vi "Launch Controller.vi"(8 "error in":errorcluster) -> ()   [LabVIEW 2016]
doc: "This VI executes continuously carrying out the current operation and responding to updates or new operations. It will often contain the timing or control code that is difficult to place directly in TeleOp. This VI generally opens all sensors and motors and isolates the rest of the robot code from knowing how the operations are carried out."
uses:
  Launch Setpoints.ctl
  Launch Operations.ctl
  <vilib>/Platform/TimedLoop/XDataNode/timing_clust.ctl
  <vilib>/Platform/TimedLoop/XDataNode/nitl_modes.ctl
  <vilib>/Platform/TimedLoop/XDataNode/wakeup.ctl
  <vilib>/Rock Robotics/Network Tables/NT Write Boolean.vi
  <vilib>/Rock Robotics/Network Tables/NT Read Boolean.vi
  <vilib>/Rock Robotics/Network Tables/NT Read Number.vi
  <vilib>/Platform/TimedLoop/XDataNode/XDataNode.xnode
  <vilib>/Platform/TimedLoop/XDataNode/XDNodeRunTimeDep.lvlib
panel:
  out "Launcher RPM":dbl=3319.8279051826034
  out "Feeder RPM":dbl=3319.8279051826034
  out "Current\nCmd":string
  # "Tip: It may be helpful to observe inputs and sensor values.\nYou may also want to display tuning or debugging controls."
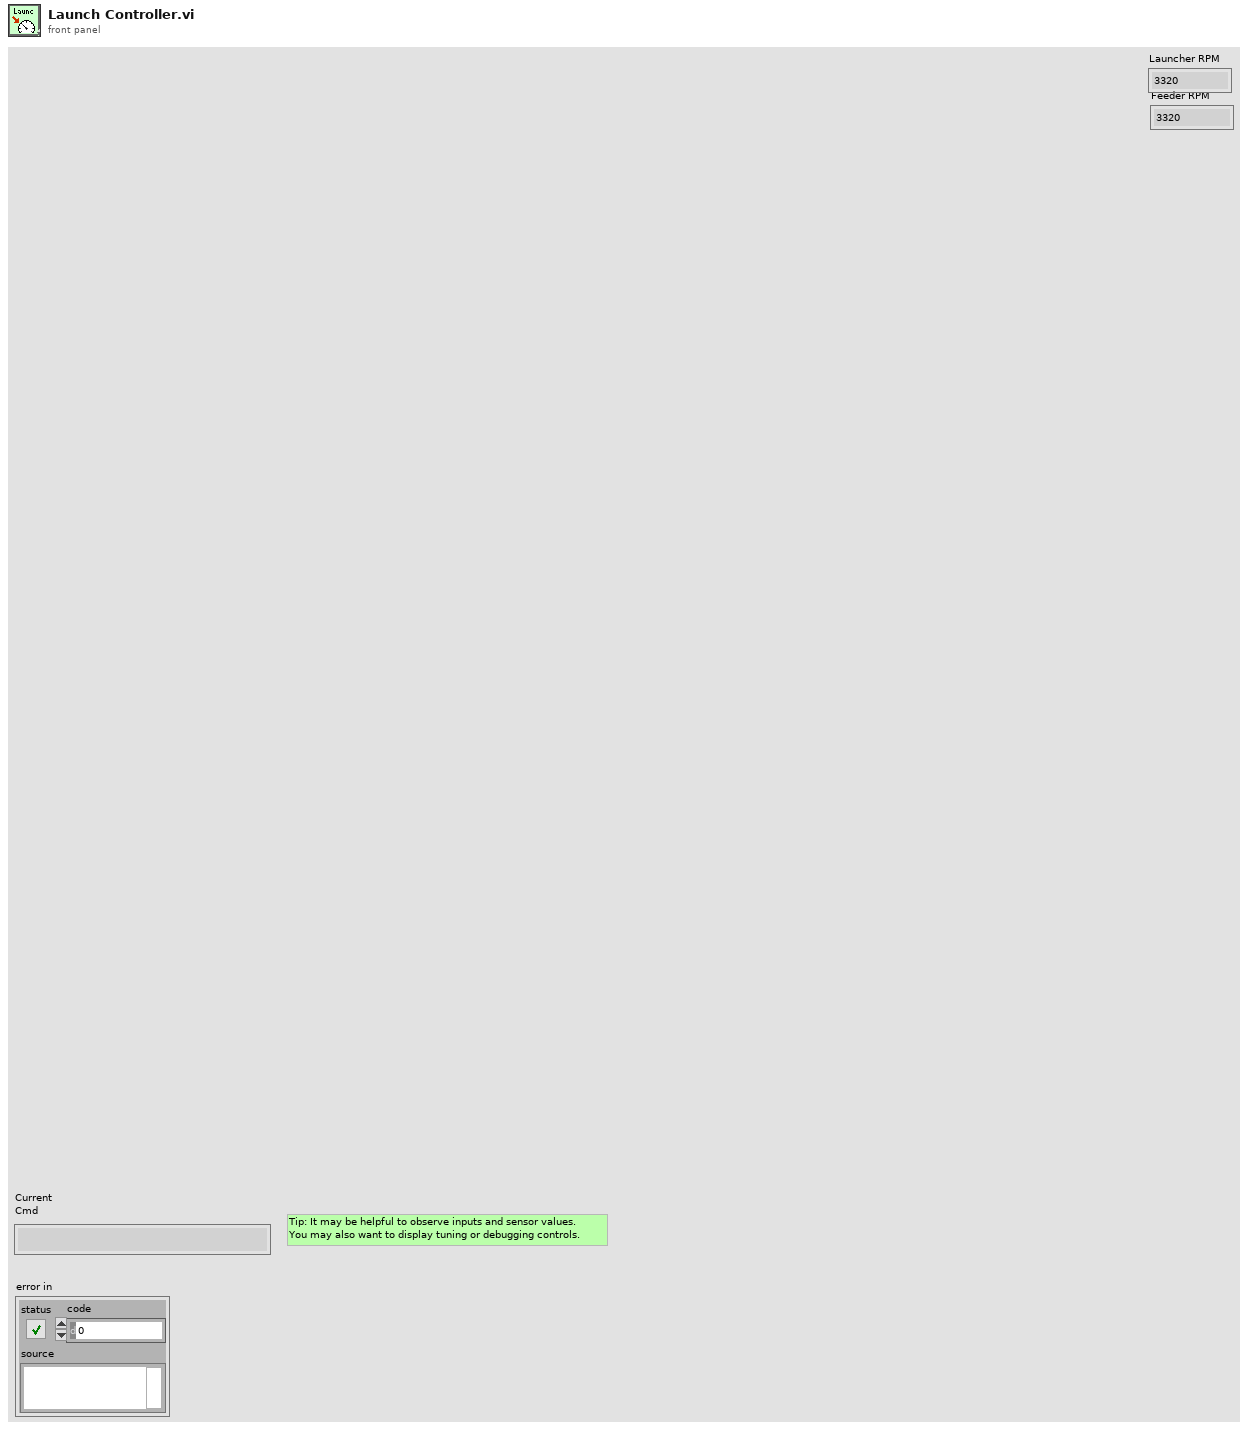
[diagram p1: front panel]
types:
  T1 = typedef "Launch Setpoints.ctl" = cluster{"Operation":T2, "Setpoint":dbl, "Duration":dbl}
  T2 = typedef "Launch Operations.ctl" = enum16{"Reserve", "Read Current", "Immediate", "Set Adgitator", "Toggle Launcher"}
  T3 = typedef "XDNodeRunTimeDep.lvlib/timing_clust.ctl" = cluster{"Expected End [f-1]":u64, "Actual End [f-1]":u64, "Finished Late? [f-1]":bool, "Expected End [i-1]":u64, "Actual End [i-1]":u64, "Finished Late? [i-1]":bool, "Expected Start [i]":u64, "Actual Start [i]":u64, "Expected Start [f]":u64, "Actual Start [f]":u64, "Source Name":string, "Structure Name":string, "Period":i64, "Deadline":i64, "Offset":i64, "Start":i64, "Priority":i32, "Timeout":i32, "Mode":T4, "Wakeup Reason":T5, "Error":errorcluster, "Source Type":string, "Secondary Source Type":string, "Global End Time":u64, "Global Start Time":u64, "Frame Duration":u64, "Iteration Duration":u64, "Assigned CPU":i32, "I/O Scan Engine Mode":u32}
  T4 = typedef "XDNodeRunTimeDep.lvlib/nitl_modes.ctl" = enum32{"No Change", "Process missed periods, maintain original phase", "Discard missed periods, maintain original phase", "Process missed periods, ignore original phase", "Discard missed periods, ignore original phase"}
  T5 = typedef "XDNodeRunTimeDep.lvlib/wakeup.ctl" = enum32{"Normal", "Aborted", "Asynchronous wakeup", "Timing source error", "Timed loop error", "Timeout"}
  T6 = typedef "WPI_MotorControlDeviceRef.ctl" = cluster{"DeviceStatus":errorcluster, "Type":T7, "PWM":cluster{"PWM Channel":T8, "DeadBand":T9}, "CAN":cluster{"Device Number":u8, "SetOutput VI Ref":variant, "GetOutput VI Ref":variant, "Enable VI Ref":variant, "Disable VI Ref":variant, "Data":variant}, "Invert":bool}
  T7 = typedef "WPI_MotorControlType.ctl" = enum16{"PWM", "CAN"}
  T8 = typedef "FPGA_DIOPWMChannel.ctl" = enum8{"PWM 0", "PWM 1", "PWM 2", "PWM 3", "PWM 4", "PWM 5", "PWM 6", "PWM 7", "PWM 8", "PWM 9", "PWM MXP 0", "PWM MXP 1", "PWM MXP 2", "PWM MXP 3", "PWM MXP 4", "PWM MXP 5", "PWM MXP 6", "PWM MXP 7", "PWM MXP 8", "PWM MXP 9", "Invalid"}
  T9 = typedef "WPI_PWMDeadband.ctl" = cluster{"Name":string, "maxPositivePwm":i32, "minPositivePwm":i32, "centerPwm":i32, "maxNegativePwm":i32, "minNegativePwm":i32, "angularRange":u16}
  T10 = typedef "Command Status Info.ctl" = cluster{"Name":string, "Status":T11, "notifier out":T12}
  T11 = typedef "Completion Status.ctl" = enum16{"Successful", "Aborted", "Incomplete"}
  T12 = typedef "Completion Notifier.ctl" = refnum<notifier>
  T13 = cluster{"Default Command":T1, "Command Timing":cluster{"Start Time (ms)":u32, "Iterations":i32}, "Command Arguments":cluster{"Command Info":T10, "Description":string, "Default Command":T1, "notifier out":refnum<notifier>, "Subsystem Name":string}}
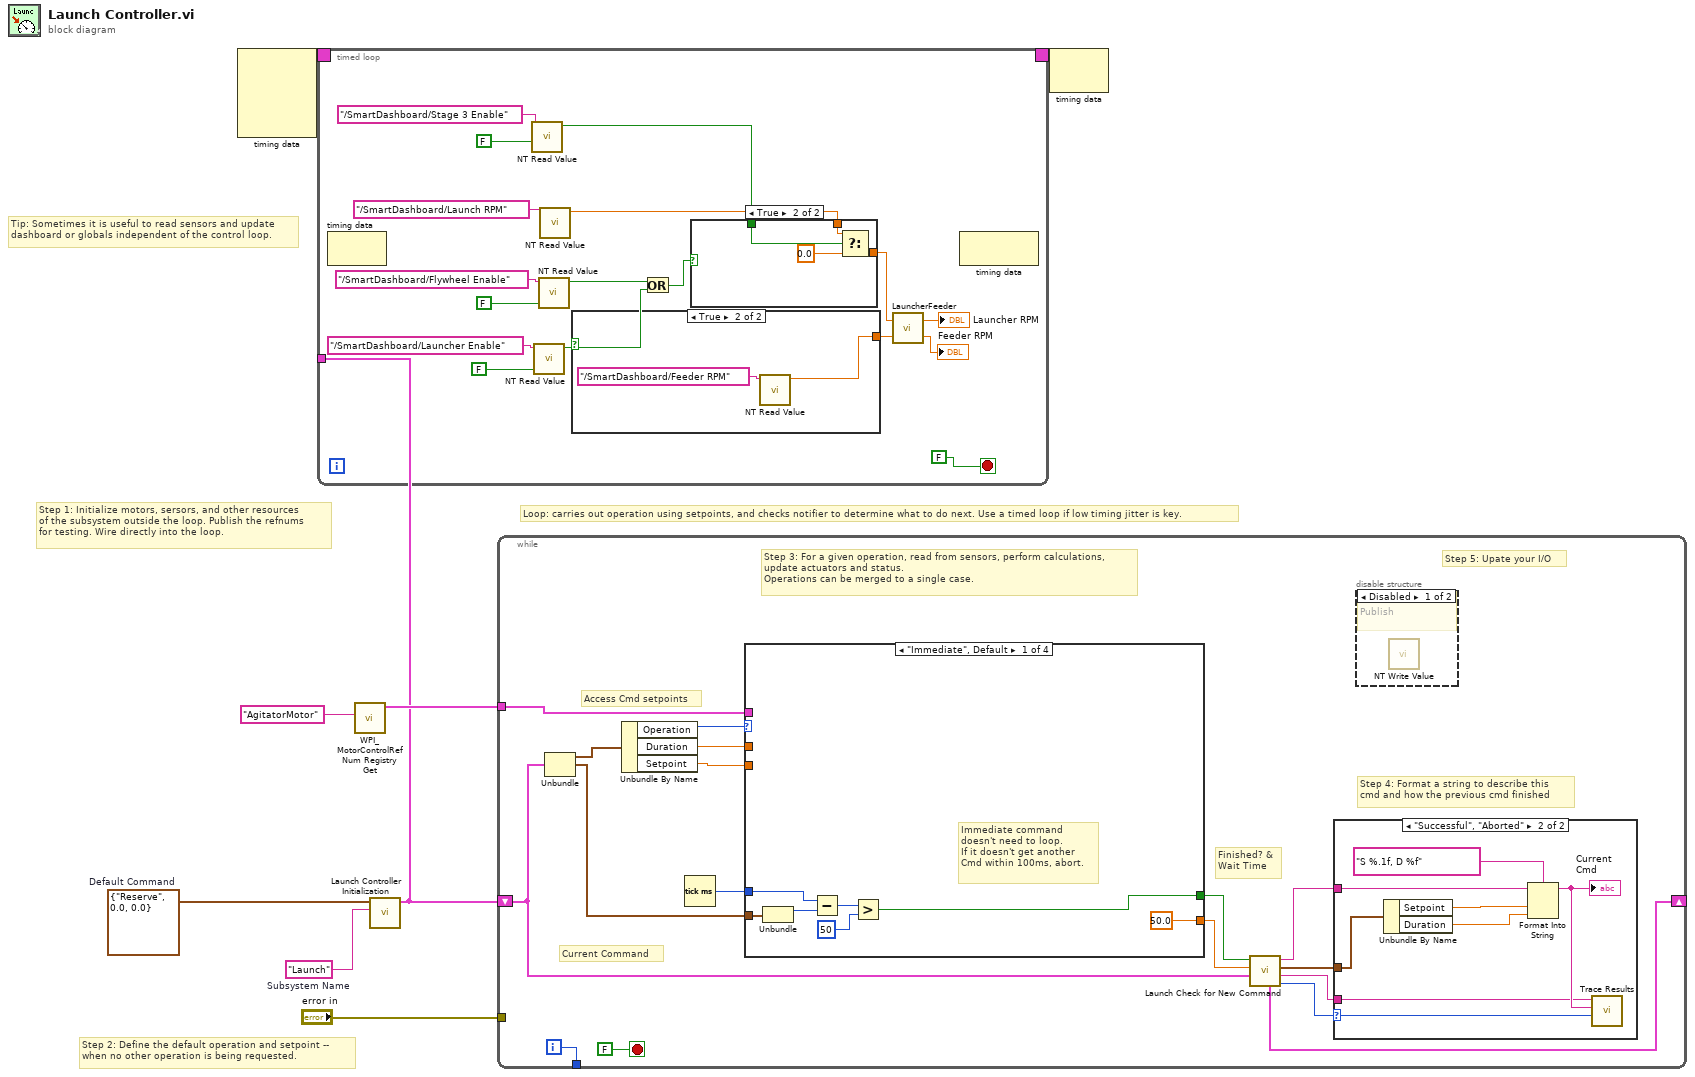
[diagram p0: block diagram]
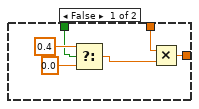
[diagram p2: hidden frame]
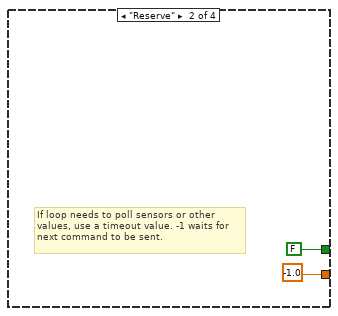
[diagram p6: hidden frame]
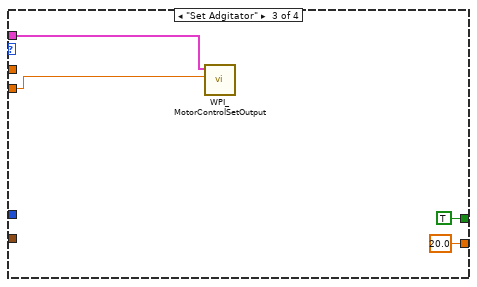
[diagram p7: hidden frame]
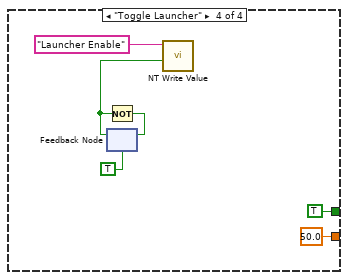
[diagram p8: hidden frame]
diagram:
  w6 = T1 {"Operation"=enum."Reserve", "Setpoint"=0.0, "Duration"=0.0}  # Default Command
  w7 = "Launch"  # Subsystem Name
  # "Tip: Sometimes it is useful to read sensors and update\ndashboard or globals independent of the control loop."
  # "Step 2: Define the default operation and setpoint --\nwhen no other operation is being requested."
  # "Step 1: Initialize motors, sersors, and other resources\nof the subsystem outside the loop. Publish the refnums\nfor testing. Wire directly into the loop."
  # "Loop: carries out operation using setpoints, and checks notifier to determine what to do next. Use a timed loop if low timing jitter is key."
  n1 = node-c288() -> (w3:T3)  [unwired: 4 in]
  n2 = call <vilib>:"WPI_MotorControlRefNum Registry Get.vi"("refnum name"="AgitatorMotor") -> ("MotorControlDevRef"=w4:T6)  [unwired: 9 in, 1 out]
  n3 = call "Launch Controller Initialization.vi"("Subsystem Name"=w7, "Default Command"=w6) -> ("Command Info"=w1:T13)  [unwired: 9 in]
  n4 = timed-loop {
    timing: w3 -> [_]
    timing-out: [_] -> w2
    tunnel: w1 -> [_]
    stop <- FALSE stop-if-true
    n5 = node-c288() -> ()  [unwired: 1 in, 1 out]
    n6 = call-poly <vilib>:"NT Read Value.vi"("Default Value"=FALSE, "Name"="/SmartDashboard/Stage 3 Enable") -> ("Boolean"=w9:bool)  [unwired: 8 in, 1 out]
    n7 = call-poly <vilib>:"NT Read Value.vi"("Default Value"=FALSE, "Name"="/SmartDashboard/Launcher Enable") -> ("Boolean"=w15:bool)  [unwired: 8 in, 1 out]
    n8 = call-poly <vilib>:"NT Read Value.vi"("Default Value"=FALSE, "Name"="/SmartDashboard/Flywheel Enable") -> ("Boolean"=w16:bool)  [unwired: 8 in, 1 out]
    n9 = call-poly <vilib>:"NT Read Value.vi"("Name"="/SmartDashboard/Launch RPM") -> ("Numeric"=w12:dbl)  [unwired: 9 in, 1 out]
    n10 = case shown="True" w15 {
      tunnel: [_ w36] -> w20
      frame False {
      }
      frame True {
        n11 = call-poly <vilib>:"NT Read Value.vi"("Name"="/SmartDashboard/Feeder RPM") -> ("Numeric"=w36:dbl)  [unwired: 9 in, 1 out]
      }
    }
    n12 = Or(x=w16, y=w15) -> (x .or. y?=w14:bool)
    n13 = case shown="True" w14 {
      tunnel: [w30 w34] -> w19
      tunnel: w12 -> [w31 w35]
      tunnel: w9 -> [w26 w33]
      frame False {
        n14 = Select(t=0.4 ("y"), s=w26, f=0.0) -> (s? t:f=w28:dbl)
        n15 = Multiply(x=w31, y=w28) -> (x*y=w30:dbl)
      }
      frame True {
        n16 = Select(t=w35, s=w33, f=0.0 ("t")) -> (s? t:f=w34:dbl)
      }
    }
    n17 = call "LauncherFeeder.vi"("Target RPM Feeder"=w20, "Target RPM Launcher"=w19) -> ("Feeder RPM"=→"Feeder RPM":dbl, "Launcher RPM"=→"Launcher RPM":dbl)
    n18 = node-c288() -> ()  [unwired: 1 in, 1 out]
  }
  n19 = while {
    shift-right: [w47] -> _
    shift-left: w1 -> [w48]
    tunnel: [w55] -> _
    tunnel: "error in" -> [_]
    tunnel: w4 -> [w40]
    i -> [w55]
    stop <- FALSE stop-if-true
    # "Step 5: Upate your I/O"
    # "Step 4: Format a string to describe this\ncmd and how the previous cmd finished"
    # "Current Command"
    # "Access Cmd setpoints"
    # "Finished? &\nWait Time"
    # "Step 3: For a given operation, read from sensors, perform calculations,\nupdate actuators and status.\nOperations can be merged to a single case."
    n20 = Unbundle(w48) -> ("Default Command"=w54:T1, "Command Timing"=w50:cluster{"Start Time (ms)":u32, "Iterations":i32})  [unwired: 1 out]
    n21 = Unbundle By Name(w54) -> ("Operation"=w53:T2, "Duration"=w52:dbl, "Setpoint"=w49:dbl)
    n22 = Tick Count (ms)() -> (millisecond timer value=w51:u32)
    n23 = case shown="\"Immediate\", Default" w53 {
      tunnel: [50.0 -1.0 20.0 50.0] -> w45
      tunnel: [w65 FALSE ("ignore previous (F)") TRUE ("ignore previous (F)") TRUE ("ignore previous (F)")] -> w46
      tunnel: w50 -> [w67 _ _ _]
      tunnel: w52 -> [_ _ _ _]
      tunnel: w51 -> [w66 _ _ _]
      tunnel: w49 -> [_ _ w74 _]
      tunnel: w40 -> [_ _ w75 _]
      frame "Immediate", Default {
        # "Immediate command\ndoesn't need to loop.\nIf it doesn't get another\nCmd within 100ms, abort."
        n24 = Unbundle(w67) -> ("Start Time (ms)"=w70:u32)  [unwired: 1 out]
        n25 = Subtract(x=w66, y=w70) -> (x-y=w69:u32)
        n26 = Greater?(x=w69, y=u8 50 ("Left Motor")) -> (0:w65:bool)
      }
      frame "Reserve" {
        # "If loop needs to poll sensors or other\nvalues, use a timeout value. -1 waits for\nnext command to be sent."
      }
      frame "Set Adgitator" {
        n27 = call <vilib>:"WPI_MotorControlSetOutput.vi"("Output"=w74, "MotorControlDevRef"=w75) -> ()  [unwired: 7 in, 3 out]
      }
      frame "Toggle Launcher" {
        n28 = feedback #1(TRUE) -> (w81:bool)
        n29 = Not(x=w81) -> (.not. x?=w80:bool)
        n30 = feedback-in #1(w80) -> ()
        n31 = call-poly <vilib>:"NT Write Value.vi"("Boolean"=w81, "Name"="Launcher Enable") -> ()  [unwired: 9 in, 1 out]
      }
    }
    n32 = call "Launch Check for New Command.vi"("Current Command"=w48, "Wait time (ms)"=w45, "Finished?"=w46) -> ("Completion"=w41:T11, "Subsystem Name"=w42:string, "Current Command"=w43:T1, "Initial Trace String"=w44:string, "NextCommand"=w47:T13)  [unwired: 4 in]
    n33 = case shown="\"Successful\", \"Aborted\"" w41 {
      selector: w41 -> [_ w64]
      tunnel: w44 -> [_ w60]
      tunnel: w43 -> [_ w61]
      tunnel: w42 -> [_ w57]
      frame "Incomplete", Default {
        # "Continuing current command"
      }
      frame "Successful", "Aborted" {
        # "Report and setup for next command"
        n34 = Unbundle By Name(w61) -> ("Setpoint"=w63:dbl, "Duration"=w58:dbl)
        n35 = Format Into String(format string="S %.1f, D %f", initial string=w60, w63, w58) -> (resulting string=w59:string)  [unwired: 1 in, 1 out]
        "Current\nCmd" <- w59
        n36 = call <vilib>:"Trace Results.vi"("Status of previous command"=w64, "Description"=w59, "Subsystem"=w57) -> ()  [unwired: 9 in]
      }
    }
    n37 = disable-structure shown="Disabled" {
      frame Disabled {
        # "Publish"
        n38 = call-poly <vilib>:"NT Write Value.vi"() -> ()  [unwired: 11 in, 1 out]
      }
      frame Enabled {
      }
    }
  }
  n39 = node-c288(w2) -> ()  [unwired: 1 out]
